vi "FINAL PELLET .vi"() -> ()   [LabVIEW 2016]
uses:
  <vilib>/NXT/NXT Controls/ConnectionType.ctl
  <vilib>/NXT/Block Support/NXT_OutputPort.ctl
  <vilib>/NXT/Block Support/NXT_InputPort.ctl
  <vilib>/NXT/Dual Mode Library/Sensors/EV3_Color_Color.vi
  <vilib>/NXT/NXTIO Xnodes/NXTIONodeSubVIs/NXTMotorRunDistance.vi
  <vilib>/NXT/Dual Mode Library/Waits/Wait_Num.vi
  <vilib>/NXT/NXTIO Xnodes/NXTIONodeSubVIs/NXTStopMotors.vi
  <vilib>/NXT/Dual Mode Library/Sensors/EV3_Color_RGB.vi
  <vilib>/NXT/NXTIO Xnodes/AddressXNode/NXTIOAddress.xnode
  <vilib>/NXT/Subs/LVHSConnector.ctl
  <vilib>/NXT/NXTIO Xnodes/NXTIOXNode/NXTIO.xnode
  <vilib>/NXT/LegoClasses/BrickReference/BrickReference.lvclass
panel:
  out "Material Binary":string
  out "Type Binary":string
  out "Material":dbl[](array[numeric])
  out "Type":dbl[](array[numeric])
  in  "Time 2":dbl
  in  "Pause":dbl
  in  "Time 1":dbl
  out "Type":string[](array[string])
  out "Type Binary":string[](array[string])
  out "Material":string[](array[string])
  out "Material Binary":string[](array[string])
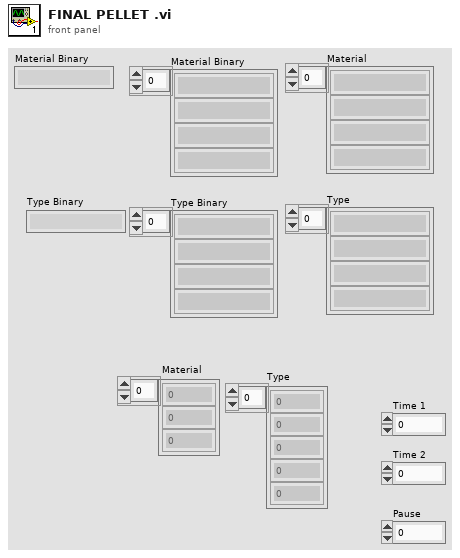
[diagram p1: front panel]
types:
  T1 = typedef "ConnectionType.ctl" = enum16{"Bluetooth", "USB", "WiFi"}
  T2 = typedef "LVHSConnector.ctl" = refnum<class "BrickReference.lvclass">
  T3 = typedef "NXT_InputPort.ctl" = u32
  T4 = typedef "ColorSensorColors.ctl" = enum16{"No Color", "Black", "Blue", "Green", "Yellow", "Red", "White", "Brown"}
  T5 = typedef "NXT_OutputPort.ctl" = u8
  T6 = cluster{"[0]":string, "[1]":string, "[2]":string, "[3]":string, "[4]":string, "[5]":string, "[6]":string, "[7]":string, "[8]":string}
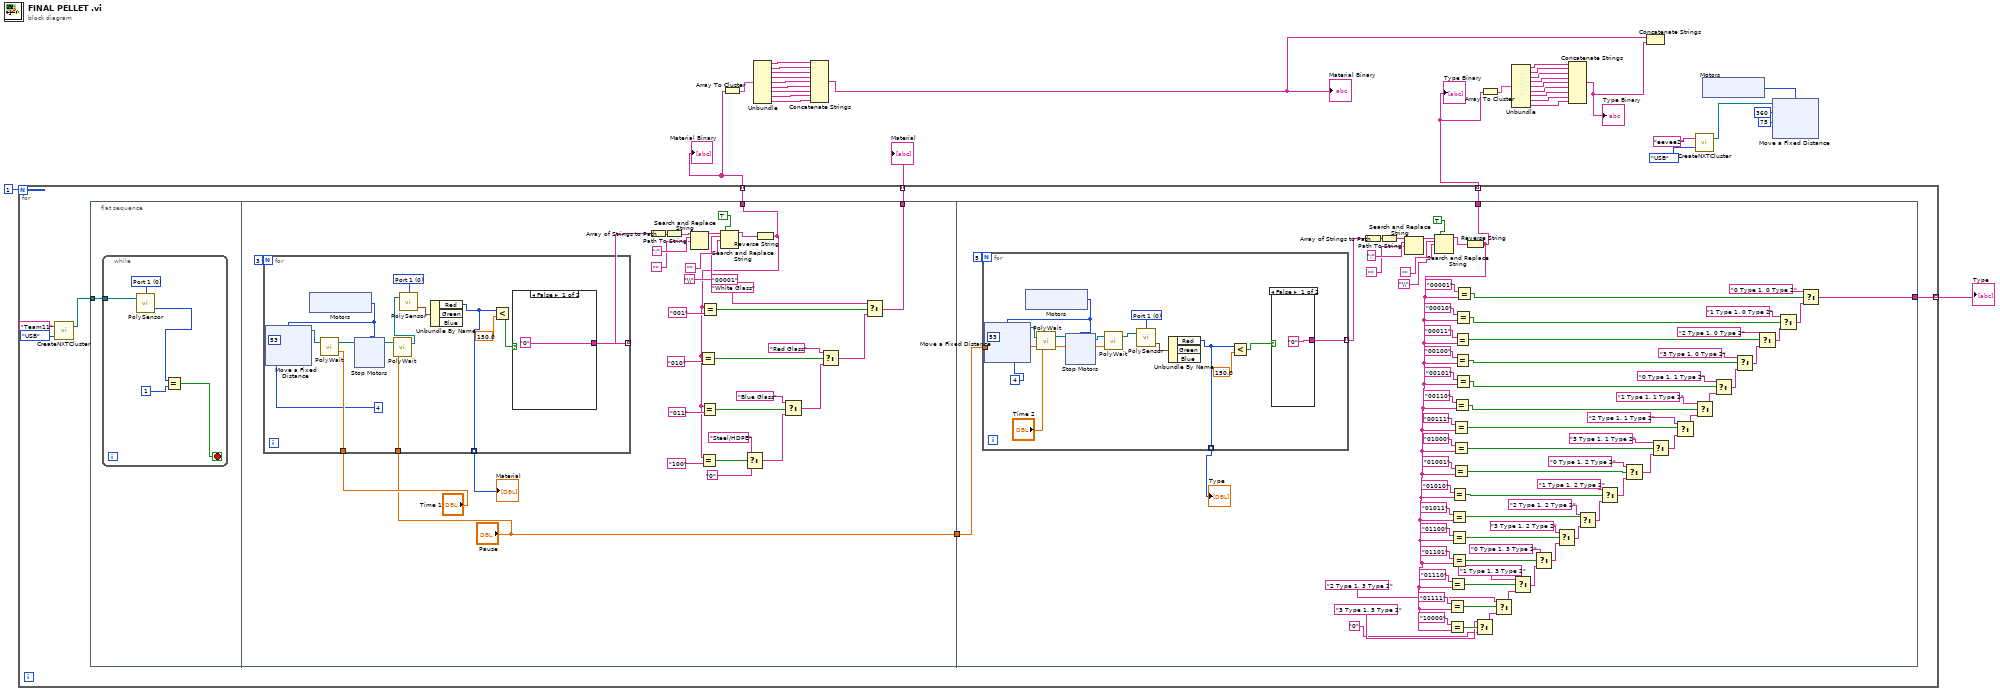
[diagram p0: block diagram]
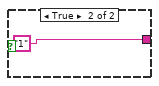
[diagram p2: hidden frame]
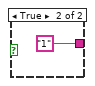
[diagram p3: hidden frame]
diagram:
  n1 = for {
    N: 1 -> [_]
    tunnel: [w41] -> w32 mode=indexing
    tunnel: [w40] -> w31 mode=indexing
    tunnel: [w39] -> w30 mode=indexing
    tunnel: [w38] -> w9 mode=indexing
    n2 = call <vilib>:"CreateNXTCluster.vi"("Connection Type"=ConnectionType."USB", "NXT/EV3 name"="Team11") -> ("NXT/EV3"=w34:T2)  [unwired: 2 in]
    n3 = flat-sequence {
      tunnel: w34 -> [w42]
      tunnel: [w64] -> w41
      tunnel: [w50] -> w38
      tunnel: ["Pause"] -> w37
      tunnel: [w125] -> w40
      tunnel: [w113] -> w39
      tunnel: w37 -> [w117]
      frame #0 {
        n4 = while {
          tunnel: w42 -> [w43]
          stop <- w45 stop-if-true
          w44 = T3 0 items=["Port 1", "Port 2", "Port 3", "Port 4"] ("Port (Port 1)")
          n5 = call-poly <vilib>:"PolySensor.vi"("NXT/EV3"=w43, "Port (Port 1)"=w44) -> ("Detected Color"=w47:T4)  [unwired: 1 in, 1 out]
          n6 = Equal?(x=w47, y=1) -> (x = y?=w45:bool)
        }
      }
      frame #1 {
        (unwired) "00001"
        n7 = for {
          N: 3 -> [_]
          tunnel: [w94] -> w52 mode=indexing
          tunnel: "Time 1" -> [w92]
          tunnel: "Pause" -> [w90]
          tunnel: [w85] -> w53 mode=indexing
          w89 = T3 0 items=["Port 1", "Port 2", "Port 3", "Port 4"] ("Port (Port 1)")
          n8 = xnode "Motors"() -> ("Motor"=w81:T5)
          n9 = xnode "Move a Fixed Distance"("Speed 1"=4, "Distance 1"=53, "Motors"=w81) -> ("NXT/EV3"=w82:T2)  [unwired: 1 in]
          n10 = call-poly <vilib>:"PolyWait.vi"("Time (1 sec)"=w92, "NXT/EV3"=w82) -> ("NXT/EV3"=w93:T2)  [unwired: 2 in]
          n11 = xnode "Stop Motors"("Motors"=w81, "NXT/EV3"=w93) -> ("NXT/EV3"=w91:T2)
          n12 = call-poly <vilib>:"PolyWait.vi"("Time (1 sec)"=w90, "NXT/EV3"=w91) -> ("NXT/EV3"=w86:T2)  [unwired: 2 in]
          n13 = call-poly <vilib>:"PolySensor.vi"("NXT/EV3"=w86, "Port (Port 1)"=w89) -> ("RGB Color"=w84:cluster{"Red":u8, "Green":u8, "Blue":u8})  [unwired: 1 in, 1 out]
          n14 = Unbundle By Name(w84) -> ("Red"=w85:u8)  [unwired: 2 out]
          n15 = Less?(x=w85, y=150.0) -> (x < y?=w87:bool)
          n16 = case shown="False" w87 {
            tunnel: ["0" "1"] -> w94
            frame False {
            }
            frame True {
            }
          }
        }
        "Material" <- w53
        n17 = Array of Strings to Path(0:w52) -> (2:w63:path)  [unwired: 1 in]
        n18 = Path To String(path=w63) -> (string=w62:string)
        n19 = Search and Replace String(input string=w62, search string=":", replace string="") -> (result string=w59:string)  [unwired: 5 in, 3 out]
        n20 = Search and Replace String(replace all?=TRUE, input string=w59, search string="\\", replace string="") -> (result string=w51:string)  [unwired: 4 in, 3 out]
        n21 = Reverse String(1:w51) -> (0:w50:string)
        n22 = Equal?(x=w50, y="010") -> (x = y?=w49:bool)
        n23 = Equal?(x=w50, y="100") -> (x = y?=w68:bool)
        n24 = Equal?(x=w50, y="011") -> (x = y?=w69:bool)
        n25 = Equal?(x=w50, y="001") -> (x = y?=w48:bool)
        n26 = Select(t="Steel/HDPE", s=w68, f="0") -> (s? t:f=w67:string)
        n27 = Select(t="Blue Glass", s=w69, f=w67) -> (s? t:f=w71:string)
        n28 = Select(t="Red Glass", s=w49, f=w71) -> (s? t:f=w73:string)
        n29 = Select(t="White Glass", s=w48, f=w73) -> (s? t:f=w64:string)
      }
      frame #2 {
        n30 = for {
          N: 5 -> [_]
          tunnel: [w205] -> w115 mode=indexing
          tunnel: w117 -> [w203]
          tunnel: [w196] -> w116 mode=indexing
          w206 = T3 0 items=["Port 1", "Port 2", "Port 3", "Port 4"] ("Port (Port 1)")
          n31 = xnode "Motors"() -> ("Motor"=w193:T5)
          n32 = xnode "Move a Fixed Distance"("Speed 1"=4, "Distance 1"=53, "Motors"=w193) -> ("NXT/EV3"=w194:T2)  [unwired: 1 in]
          n33 = call-poly <vilib>:"PolyWait.vi"("Time (1 sec)"="Time 2", "NXT/EV3"=w194) -> ("NXT/EV3"=w204:T2)  [unwired: 2 in]
          n34 = xnode "Stop Motors"("Motors"=w193, "NXT/EV3"=w204) -> ("NXT/EV3"=w202:T2)
          n35 = call-poly <vilib>:"PolyWait.vi"("Time (1 sec)"=w203, "NXT/EV3"=w202) -> ("NXT/EV3"=w201:T2)  [unwired: 2 in]
          n36 = call-poly <vilib>:"PolySensor.vi"("NXT/EV3"=w201, "Port (Port 1)"=w206) -> ("RGB Color"=w199:cluster{"Red":u8, "Green":u8, "Blue":u8})  [unwired: 1 in, 1 out]
          n37 = Unbundle By Name(w199) -> ("Red"=w196:u8)  [unwired: 2 out]
          n38 = Less?(x=w196, y=150.0) -> (x < y?=w197:bool)
          n39 = case shown="False" w197 {
            tunnel: ["0" "1"] -> w205
            frame False {
            }
            frame True {
            }
          }
        }
        "Type" <- w116
        n40 = Array of Strings to Path(0:w115) -> (2:w190:path)  [unwired: 1 in]
        n41 = Path To String(path=w190) -> (string=w124:string)
        n42 = Search and Replace String(input string=w124, search string=":", replace string="") -> (result string=w121:string)  [unwired: 5 in, 3 out]
        n43 = Search and Replace String(replace all?=TRUE, input string=w121, search string="\\", replace string="") -> (result string=w114:string)  [unwired: 4 in, 3 out]
        n44 = Reverse String(1:w114) -> (0:w113:string)
        n45 = Equal?(x="01111", y=w113) -> (x = y?=w172:bool)
        n46 = Equal?(x="10000", y=w113) -> (x = y?=w173:bool)
        n47 = Equal?(x="01110", y=w113) -> (x = y?=w171:bool)
        n48 = Equal?(x="01011", y=w113) -> (x = y?=w168:bool)
        n49 = Equal?(x="01100", y=w113) -> (x = y?=w169:bool)
        n50 = Equal?(x="01101", y=w113) -> (x = y?=w170:bool)
        n51 = Equal?(x="01010", y=w113) -> (x = y?=w167:bool)
        n52 = Equal?(x="01001", y=w113) -> (x = y?=w166:bool)
        n53 = Equal?(x="00111", y=w113) -> (x = y?=w164:bool)
        n54 = Equal?(x="01000", y=w113) -> (x = y?=w165:bool)
        n55 = Equal?(x="00110", y=w113) -> (x = y?=w163:bool)
        n56 = Equal?(x="00011", y=w113) -> (x = y?=w160:bool)
        n57 = Equal?(x="00100", y=w113) -> (x = y?=w161:bool)
        n58 = Equal?(x="00010", y=w113) -> (x = y?=w159:bool)
        n59 = Equal?(x="00101", y=w113) -> (x = y?=w162:bool)
        n60 = Equal?(x="00001", y=w113) -> (x = y?=w158:bool)
        n61 = Select(t="3 Type 1, 3 Type 2", s=w173, f="0") -> (s? t:f=w157:string)
        n62 = Select(t="2 Type 1, 3 Type 2", s=w172, f=w157) -> (s? t:f=w156:string)
        n63 = Select(t="1 Type 1, 3 Type 2", s=w171, f=w156) -> (s? t:f=w155:string)
        n64 = Select(t="0 Type 1, 3 Type 2", s=w170, f=w155) -> (s? t:f=w154:string)
        n65 = Select(t="3 Type 1, 2 Type 2", s=w169, f=w154) -> (s? t:f=w153:string)
        n66 = Select(t="2 Type 1, 2 Type 2", s=w168, f=w153) -> (s? t:f=w152:string)
        n67 = Select(t="1 Type 1, 2 Type 2", s=w167, f=w152) -> (s? t:f=w151:string)
        n68 = Select(t="0 Type 1, 2 Type 2", s=w166, f=w151) -> (s? t:f=w150:string)
        n69 = Select(t="3 Type 1, 1 Type 2", s=w165, f=w150) -> (s? t:f=w149:string)
        n70 = Select(t="2 Type 1, 1 Type 2", s=w164, f=w149) -> (s? t:f=w148:string)
        n71 = Select(t="1 Type 1, 1 Type 2", s=w163, f=w148) -> (s? t:f=w147:string)
        n72 = Select(t="0 Type 1, 1 Type 2", s=w162, f=w147) -> (s? t:f=w146:string)
        n73 = Select(t="3 Type 1, 0 Type 2", s=w161, f=w146) -> (s? t:f=w145:string)
        n74 = Select(t="2 Type 1, 0 Type 2", s=w160, f=w145) -> (s? t:f=w144:string)
        n75 = Select(t="1 Type 1, 0 Type 2", s=w159, f=w144) -> (s? t:f=w143:string)
        n76 = Select(t="0 Type 1, 0 Type 2", s=w158, f=w143) -> (s? t:f=w125:string)
      }
    }
  }
  "Material Binary" <- w9
  "Material" <- w32
  "Type" <- w31
  "Type Binary" <- w30
  n77 = Array To Cluster(array=w9) -> (cluster=w19:T6)
  n78 = Unbundle(w19) -> ("[0]"=w18:string, "[1]"=w17:string, "[2]"=w16:string, "[3]"=w15:string, "[4]"=w14:string, "[5]"=w13:string, "[6]"=w12:string, "[7]"=w11:string, "[8]"=w10:string)
  n79 = Concatenate Strings(w18, w17, w16, w15, w14, w13, w12, w11, w10) -> (w7:string)
  "Material Binary" <- w7
  n80 = Array To Cluster(array=w30) -> (cluster=w29:T6)
  n81 = Unbundle(w29) -> ("[0]"=w28:string, "[1]"=w27:string, "[2]"=w26:string, "[3]"=w25:string, "[4]"=w24:string, "[5]"=w23:string, "[6]"=w22:string, "[7]"=w21:string, "[8]"=w20:string)
  n82 = Concatenate Strings(w28, w27, w26, w25, w24, w23, w22, w21, w20) -> (w8:string)
  "Type Binary" <- w8
  n83 = Concatenate Strings(w7, w8) -> ()  [unwired: 1 out]
  n84 = call <vilib>:"CreateNXTCluster.vi"("Connection Type"=ConnectionType."USB", "NXT/EV3 name"="eevee2") -> ("NXT/EV3"=w1:T2)  [unwired: 2 in]
  n85 = xnode "Motors"() -> ("Motor"=w4:T5)
  n86 = xnode "Move a Fixed Distance"("Speed 1"=i8 75, "Distance 1"=360, "Motors"=w4, "NXT/EV3"=w1) -> ()  [unwired: 1 out]
